vi "Point&Path@Calculate__Parameter.vi"(1 "ParamterIn":string) -> (0 "ParamterOut":string)   [LabVIEW 2019]
panel:
  out "PointNameList":string[](array[string])
  in  "PointName":string(combo)
  in  "Confirm":bool
  # "Point&Path@Calculate\nPoint can be:  (X,Y,Z,U,.....), $PointName, $PointName[Index]\nReplace------> $Point    =  $Point A \nAppend------> $Point  <=  $Point A \nOperate----->  $Point = $Point_A +-*/ $Point_B"
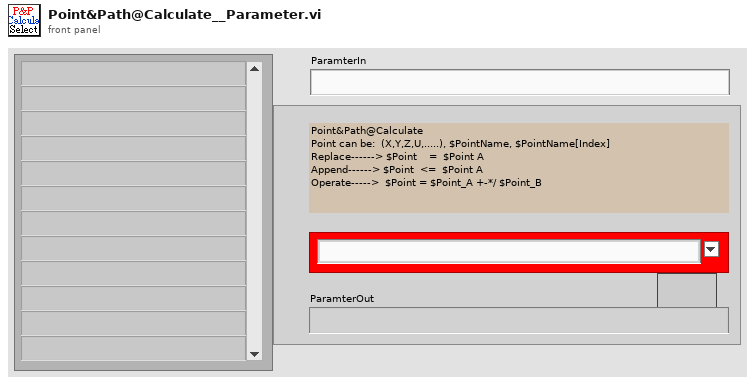
[diagram p1: front panel]
types:
  T1 = enum16{"Get", "UpdatePointS", "Init", "UpdateIndex", "GetCurrent&Index+1", "GetWithIndex", "ChkLast", "GetCurrent"}
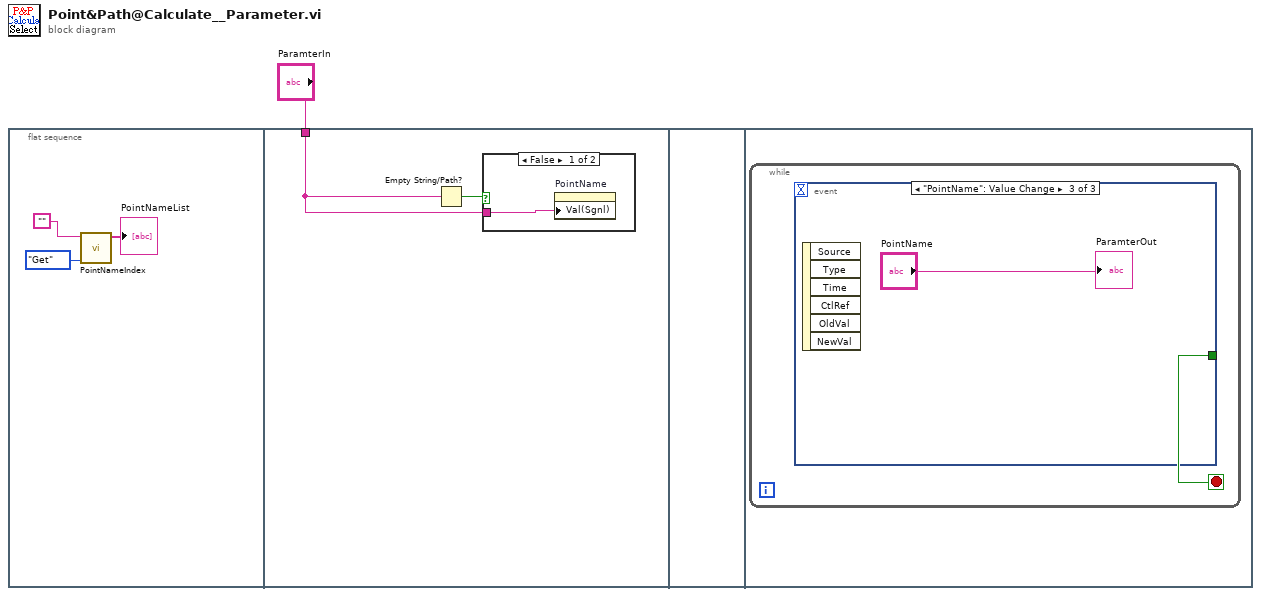
[diagram p0: block diagram]
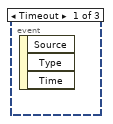
[diagram p3: hidden frame]
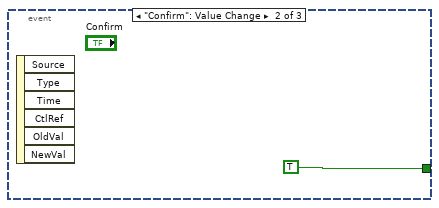
[diagram p4: hidden frame]
diagram:
  n1 = flat-sequence {
    tunnel: "ParamterIn" -> [w5]
    frame #0 {
      n2 = call "PointNameIndex.vi"("OP"=T1."Get", "PointName"="") -> ("PointNameList"=→"PointNameList":string[])  [unwired: 4 in, 5 out]
    }
    frame #1 {
      n3 = Empty String/Path?(string/path=w5) -> (empty?=w6:bool)
      n4 = case shown="False" w6 {
        tunnel: w5 -> [w7 _]
        frame False {
          n5 = property on="PointName" class="CmbBox"("Val(Sgnl)"=w7) -> ()  [unwired: 2 in, 2 out]
        }
        frame True {
        }
      }
    }
    frame #2 {
    }
    frame #3 {
      n6 = while {
        stop <- w8 stop-if-true
        n7 = event shown="[2] \"PointName\": Value Change" {
          selector: _ -> [_ _ _]
          dyn-events: _ -> [_ _ _]
          timeout: _ -> [_ _ _]
          tunnel: [_ TRUE _] -> w8
          event Timeout {
            n8 = event-data() -> ()  [unwired: 1 in, 3 out]
          }
          event "Confirm": Value Change {
            n9 = event-data() -> ()  [unwired: 1 in, 6 out]
          }
          event "PointName": Value Change {
            n10 = event-data() -> ()  [unwired: 1 in, 6 out]
            "ParamterOut" <- "PointName"
          }
        }
      }
    }
  }
